vi "Draw Actor Core UI on SubPanel.vi"(8 "error in (no error)":errorcluster, 11 "Items in":refnum<class "Items.lvclass">) -> (0 "error out":errorcluster, 3 "Items out":refnum<class "Items.lvclass">)   [LabVIEW 2020, in "Items.lvlib" / "Items.lvclass"]
uses:
  Items.lvclass
  Items.lvclass/Items.ctl
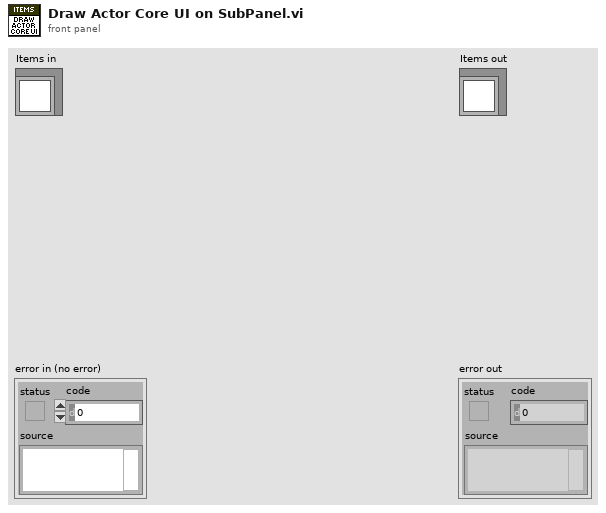
[diagram p1: front panel]
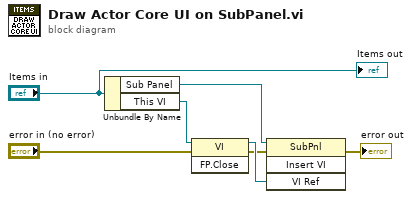
[diagram p0: block diagram]
diagram:
  n1 = Unbundle By Name("Items in") -> ("Sub Panel"=w6:refnum<vi>, "This VI"=w7:refnum<vi>)
  n2 = invoke class="VI" method="FP.Close"(reference=w7, error in="error in (no error)") -> (reference out=w5:refnum<vi>, error out=w4:errorcluster)  [unwired: 1 in, 1 out]
  n3 = invoke class="SubPnl" method="Insert VI"(reference=w6, error in=w4, "VI Ref"=w5) -> (error out=→"error out":errorcluster)  [unwired: 1 in, 3 out]
  "Items out" <- "Items in"
